vi "VerifyAcqIdle.vi"(8 "error in (no error)":errorcluster, 11 "S4GUI in":refnum<class "S4GUI.lvclass">) -> (0 "error out":errorcluster, 1 "all disabled":bool, 2 "idle":bool, 3 "S4GUI out":refnum<class "S4GUI.lvclass">)   [LabVIEW 2018, in "S4GUI.lvclass"]
uses:
  S4GUI.lvclass
  S4GUI.lvclass/S4GUI.ctl
  Acquisition/Acquisition.lvclass
  Channel/Channel.lvclass
  StateMachine/State Machine.lvclass
panel:
  # "F : 1 ou mais canal habilitado\nT :  nenhum habilitado"
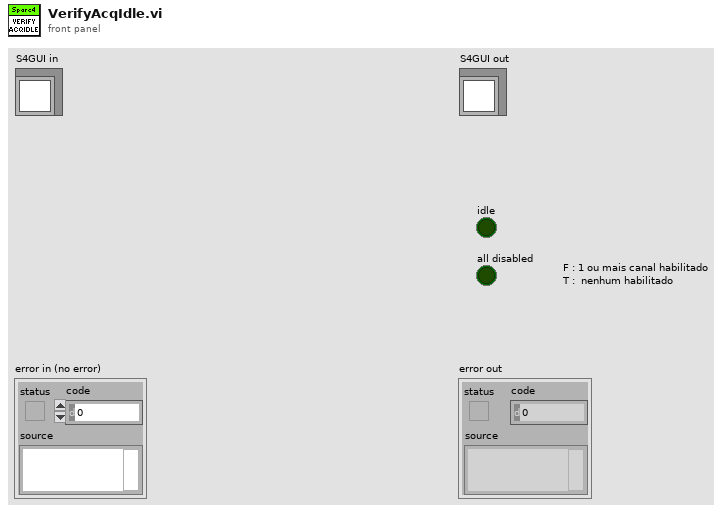
[diagram p1: front panel]
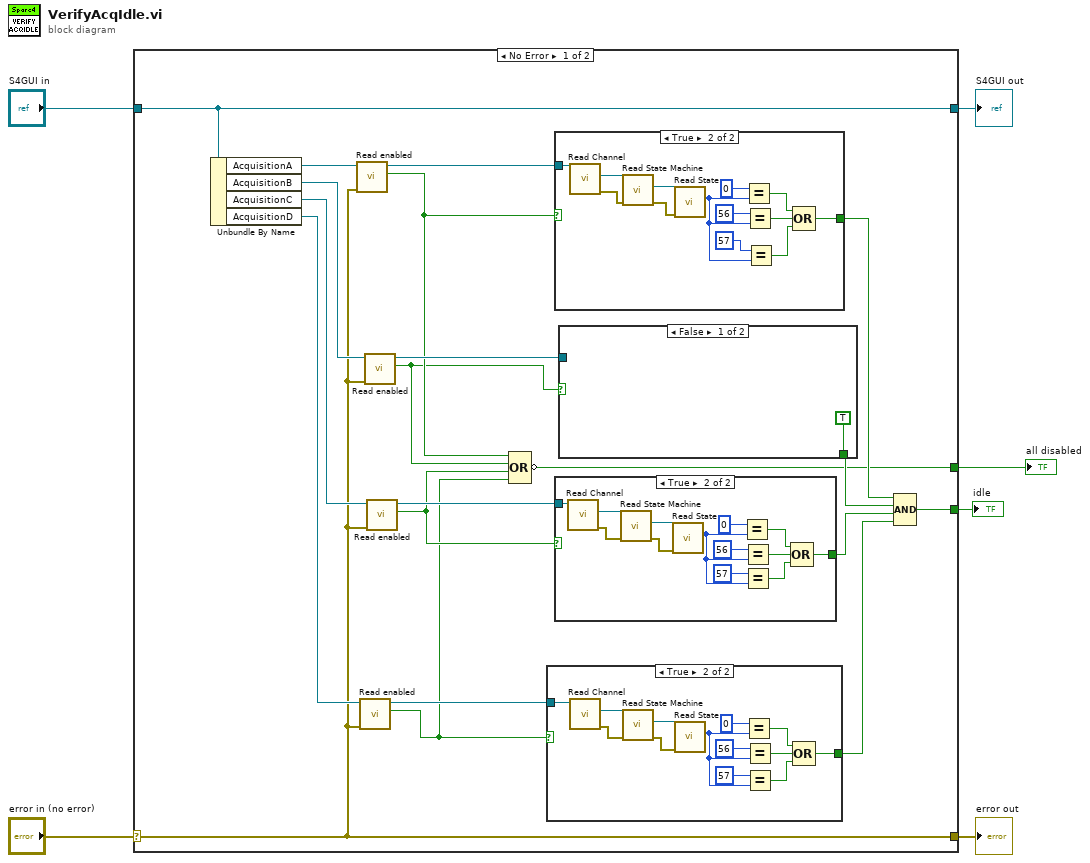
[diagram p0: block diagram]
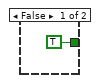
[diagram p2: hidden frame]
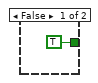
[diagram p3: hidden frame]
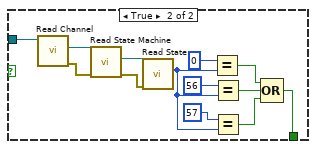
[diagram p4: hidden frame]
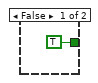
[diagram p5: hidden frame]
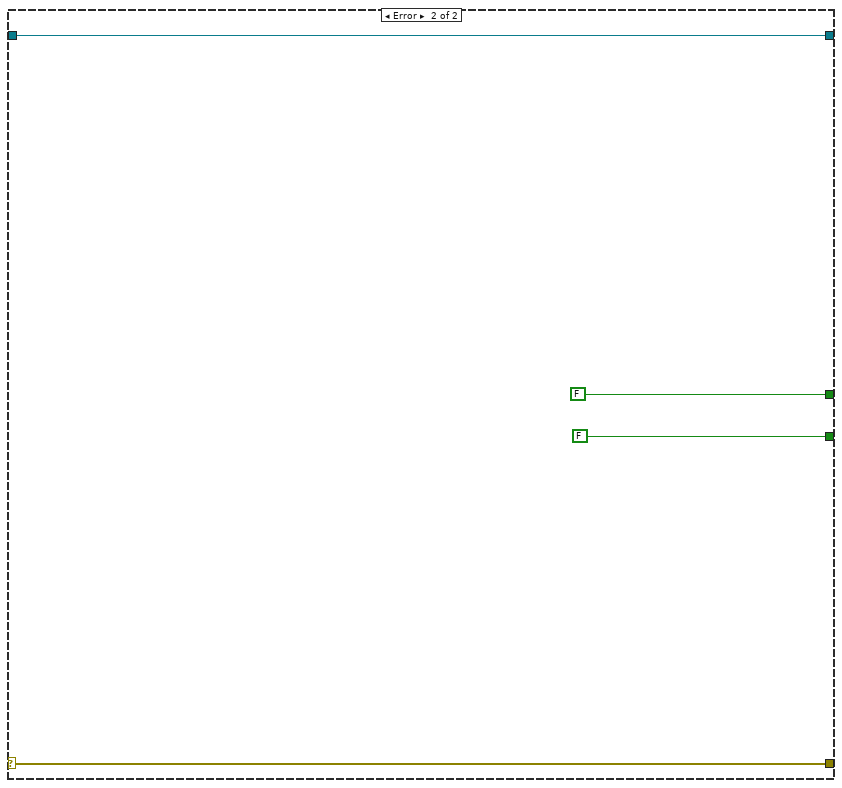
[diagram p6: hidden frame]
diagram:
  n1 = case shown="No Error" "error in (no error)" {
    selector: "error in (no error)" -> [w12 w86]
    tunnel: [w12 w86] -> w5
    tunnel: [w26 w85] -> w3
    tunnel: "S4GUI in" -> [w26 w85]
    tunnel: [w21 FALSE] -> w2
    tunnel: [w11 FALSE] -> w1
    frame No Error {
      n2 = Unbundle By Name(w26) -> ("AcquisitionA"=w20:refnum<class "Acquisition.lvclass">, "AcquisitionB"=w18:refnum<class "Acquisition.lvclass">, "AcquisitionC"=w16:refnum<class "Acquisition.lvclass">, "AcquisitionD"=w14:refnum<class "Acquisition.lvclass">)
      n3 = call-dynamic "Read enabled.vi"("error in (no error)"=w12, "Server in"=w20) -> ("enabled"=w10:bool, "Server out"=w19:refnum<class "Acquisition.lvclass">)  [unwired: 7 in, 1 out]
      n4 = call-dynamic "Read enabled.vi"("error in (no error)"=w12, "Server in"=w14) -> ("enabled"=w7:bool, "Server out"=w13:refnum<class "Acquisition.lvclass">)  [unwired: 7 in, 1 out]
      n5 = call-dynamic "Read enabled.vi"("error in (no error)"=w12, "Server in"=w18) -> ("enabled"=w9:bool, "Server out"=w17:refnum<class "Acquisition.lvclass">)  [unwired: 7 in, 1 out]
      n6 = call-dynamic "Read enabled.vi"("error in (no error)"=w12, "Server in"=w16) -> ("enabled"=w8:bool, "Server out"=w15:refnum<class "Acquisition.lvclass">)  [unwired: 7 in, 1 out]
      n7 = Compound Arithmetic op=OR(w10, w9, w8, w7) -> (invert w11:bool)
      n8 = case shown="True" w7 {
        tunnel: w13 -> [_ w31]
        tunnel: [TRUE w30] -> w22
        frame False {
        }
        frame True {
          n9 = call-dynamic "Read Channel.vi"("Acquisition in"=w31) -> ("error out"=w29:errorcluster, "Channel.lvclass"=w36:refnum<class "Channel.lvclass">)  [unwired: 8 in, 1 out]
          n10 = call-dynamic "Read State Machine.vi"("error in (no error)"=w29, "Device in"=w36) -> ("error out"=w28:errorcluster, "State Machine.lvclass"=w35:refnum<class "State Machine.lvclass">)  [unwired: 7 in, 1 out]
          n11 = call-dynamic "Read State.vi"("error in (no error)"=w28, "State Machine in"=w35) -> ("State"=w34:i32)  [unwired: 7 in, 2 out]
          n12 = Equal?(x=0, y=w34) -> (x = y?=w39:bool)
          n13 = Equal?(x=56, y=w34) -> (x = y?=w38:bool)
          n14 = Equal?(x=57, y=w34) -> (x = y?=w37:bool)
          n15 = Compound Arithmetic op=OR(w39, w38, w37) -> (w30:bool)
        }
      }
      n16 = case shown="True" w10 {
        tunnel: [TRUE w78] -> w25
        tunnel: w19 -> [_ w77]
        frame False {
        }
        frame True {
          n17 = call-dynamic "Read Channel.vi"("Acquisition in"=w77) -> ("error out"=w71:errorcluster, "Channel.lvclass"=w76:refnum<class "Channel.lvclass">)  [unwired: 8 in, 1 out]
          n18 = call-dynamic "Read State Machine.vi"("error in (no error)"=w71, "Device in"=w76) -> ("error out"=w70:errorcluster, "State Machine.lvclass"=w75:refnum<class "State Machine.lvclass">)  [unwired: 7 in, 1 out]
          n19 = call-dynamic "Read State.vi"("error in (no error)"=w70, "State Machine in"=w75) -> ("State"=w74:i32)  [unwired: 7 in, 2 out]
          n20 = Equal?(x=0, y=w74) -> (x = y?=w81:bool)
          n21 = Equal?(x=56, y=w74) -> (x = y?=w80:bool)
          n22 = Equal?(x=57, y=w74) -> (x = y?=w79:bool)
          n23 = Compound Arithmetic op=OR(w81, w80, w79) -> (w78:bool)
        }
      }
      n24 = case shown="True" w8 {
        tunnel: w15 -> [_ w45]
        tunnel: [TRUE w44] -> w23
        frame False {
        }
        frame True {
          n25 = call-dynamic "Read Channel.vi"("Acquisition in"=w45) -> ("error out"=w43:errorcluster, "Channel.lvclass"=w50:refnum<class "Channel.lvclass">)  [unwired: 8 in, 1 out]
          n26 = call-dynamic "Read State Machine.vi"("error in (no error)"=w43, "Device in"=w50) -> ("error out"=w42:errorcluster, "State Machine.lvclass"=w49:refnum<class "State Machine.lvclass">)  [unwired: 7 in, 1 out]
          n27 = call-dynamic "Read State.vi"("error in (no error)"=w42, "State Machine in"=w49) -> ("State"=w48:i32)  [unwired: 7 in, 2 out]
          n28 = Equal?(x=0, y=w48) -> (x = y?=w53:bool)
          n29 = Equal?(x=56, y=w48) -> (x = y?=w52:bool)
          n30 = Equal?(x=57, y=w48) -> (x = y?=w51:bool)
          n31 = Compound Arithmetic op=OR(w53, w52, w51) -> (w44:bool)
        }
      }
      n32 = case shown="False" w9 {
        tunnel: w17 -> [_ w59]
        tunnel: [TRUE w58] -> w24
        frame False {
        }
        frame True {
          n33 = call-dynamic "Read Channel.vi"("Acquisition in"=w59) -> ("error out"=w57:errorcluster, "Channel.lvclass"=w64:refnum<class "Channel.lvclass">)  [unwired: 8 in, 1 out]
          n34 = call-dynamic "Read State Machine.vi"("error in (no error)"=w57, "Device in"=w64) -> ("error out"=w56:errorcluster, "State Machine.lvclass"=w63:refnum<class "State Machine.lvclass">)  [unwired: 7 in, 1 out]
          n35 = call-dynamic "Read State.vi"("error in (no error)"=w56, "State Machine in"=w63) -> ("State"=w62:i32)  [unwired: 7 in, 2 out]
          n36 = Equal?(x=0, y=w62) -> (x = y?=w67:bool)
          n37 = Equal?(x=56, y=w62) -> (x = y?=w66:bool)
          n38 = Equal?(x=57, y=w62) -> (x = y?=w65:bool)
          n39 = Compound Arithmetic op=OR(w67, w66, w65) -> (w58:bool)
        }
      }
      n40 = Compound Arithmetic op=AND(w25, w24, w23, w22) -> (w21:bool)
    }
    frame Error {
    }
  }
  "error out" <- w5
  "S4GUI out" <- w3
  "idle" <- w2
  "all disabled" <- w1
